vi "Network.vi"() -> ()   [LabVIEW 2018]
panel:
  out "Pressure Sensor 4":bool
  out "Temperature Sensor 4":bool
  out "Level Sensor 4":bool
  out "Pressure Sensor 3":bool
  out "Temperature Sensor 3":bool
  out "Level Sensor 3":bool
  out "Pressure Sensor 2":bool
  out "Temperature Sensor 2":bool
  out "Level Sensor 2":bool
  out "Pressure Sensor":bool
  out "Temperature Sensor":bool
  out "Level Sensor":bool
  out "Controller":bool
  out "Status":i32(ring) items=["Success"=0, "DestinationNetworkUnreachable"=11002, "DestinationHostUnreachable"=11003, "DestinationProhibited, DestinationProtocolUnreachable"=11004, "DestinationPortUnreachable"=11005, "NoResources"=11006, "BadOption"=11007, "HardwareError"=11008, "PacketTooBig"=11009, "TimedOut"=11010, "BadRoute"=11012, "TtlExpired"=11013, "TtlReassemblyTimeExceeded"=11014, "ParameterProblem"=11015, "SourceQuench"=11016, "BadDestination"=11018, "DestinationUnreachable"=11040, "TimeExceeded"=11041, "BadHeader"=11042, "UnrecognizedNextHeader"=11043, "IcmpError"=11044, "DestinationScopeMismatch"=11045, "Unknown"=-1]
  in  "Ping Button":bool
  in  "stop 2":bool
  in  "stop":bool
  # "Connected Devices"
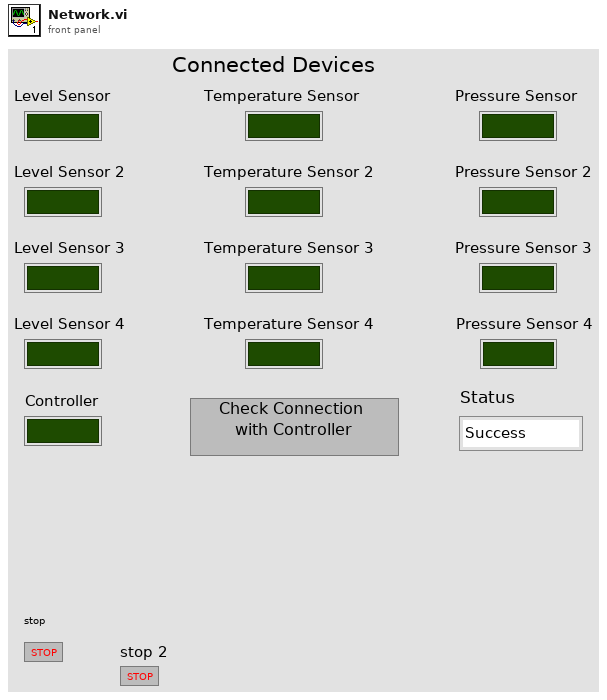
[diagram p1: front panel]
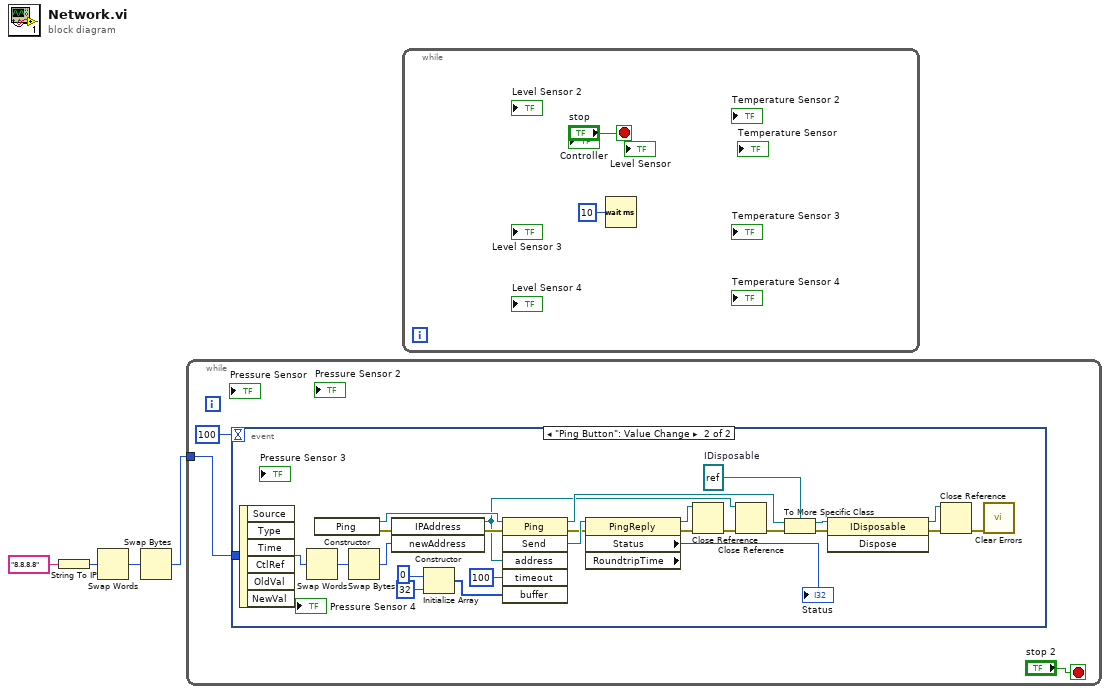
[diagram p0: block diagram]
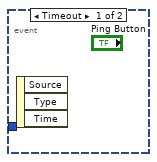
[diagram p2: hidden frame]
diagram:
  n1 = String To IP(1:"8.8.8.8" ("name")) -> (0:w3:u32)
  n2 = Swap Words(1:w3) -> (0:w4:u32)
  n3 = Swap Bytes(anything=w4) -> (byte swapped=w1:u32)
  n4 = while {
    tunnel: w1 -> [w5]
    stop <- "stop 2" stop-if-true
    n5 = event shown="[1] \"Ping Button\": Value Change" {
      selector: _ -> [_ _]
      dyn-events: _ -> [_ _]
      timeout: 100 -> [_ _]
      tunnel: w5 -> [_ w13]
      event Timeout {
        n6 = event-data() -> ()  [unwired: 1 in, 3 out]
      }
      event "Ping Button": Value Change {
        w14 = refnum<k24> refnum  # IDisposable
        n7 = event-data() -> ()  [unwired: 1 in, 6 out]
        n8 = Swap Words(1:w13) -> (0:w26:u32)
        n9 = constructor class="Ping"() -> (reference out=w30:refnum<k24>, error out=w29:errorcluster)  [unwired: 3 in, 1 out]
        n10 = Swap Bytes(anything=w26) -> (byte swapped=w27:u32)
        n11 = constructor class="IPAddress"(error in=w29, "newAddress"=w27) -> (reference out=w21:refnum<k24>, error out=w28:errorcluster)  [unwired: 2 in, 2 out]
        n12 = Initialize Array(0 ("dimension size"), 32 ("dimension size")) -> (w8:i32[])
        n13 = invoke class="Ping" method="Send"(reference=w30, error in=w28, "address"=w21, "timeout"=100, "buffer"=w8) -> (reference out=w25:refnum<k24>, error out=w31:errorcluster, "Send"=w32:refnum<k24>)  [unwired: 1 in, 3 out]
        n14 = property class="PingReply" props=["Status", "RoundtripTime"](reference=w32, error in=w31) -> (reference out=w24:refnum<k24>, error out=w23:errorcluster, "Status"=→"Status":i32)  [unwired: 1 out]
        n15 = Close Reference(reference=w24, error in (no error)=w23) -> (error out=w22:errorcluster)
        n16 = Close Reference(reference=w21, error in (no error)=w22) -> (error out=w20:errorcluster)
        n17 = To More Specific Class(target class=w14, reference=w25, error in=w20) -> (specific class reference=w19:refnum<k24>, error out=w18:errorcluster)
        n18 = invoke class="IDisposable" method="Dispose"(reference=w19, error in=w18) -> (reference out=w16:refnum<k24>, error out=w17:errorcluster)  [unwired: 1 in, 1 out]
        n19 = Close Reference(reference=w16, error in (no error)=w17) -> (error out=w15:errorcluster)
        n20 = call <vilib>:"Clear Errors.vi"("error in (no error)"=w15) -> ()  [unwired: 5 in, 2 out]
      }
    }
  }
  n21 = while {
    stop <- "stop" stop-if-true
    n22 = Wait (ms)(milliseconds to wait=u32 10) -> ()  [unwired: 1 out]
  }
